vi "Histerisis.vi"() -> ()   [LabVIEW 2020]
uses:
  <vilib>/numeric/Random Number (Range) U64.vi
  <vilib>/numeric/sub_Random U32.vi
panel:
  in  "stop":bool
  out "XY Graph 2":cluster{i32, "number":u64}[](graph)
  in  "Minimo 2":u64
  in  "Maximo 2":u64
  out "Señal 2":bool
  out "Numero 2":u64
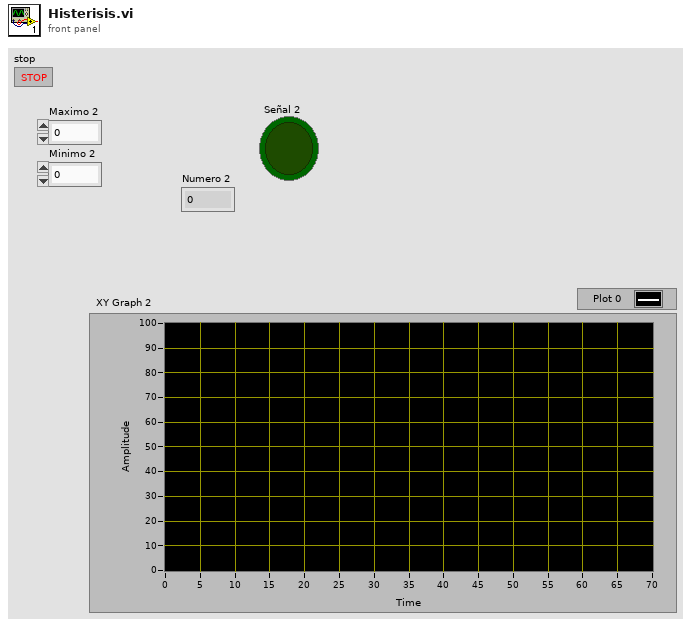
[diagram p1: front panel]
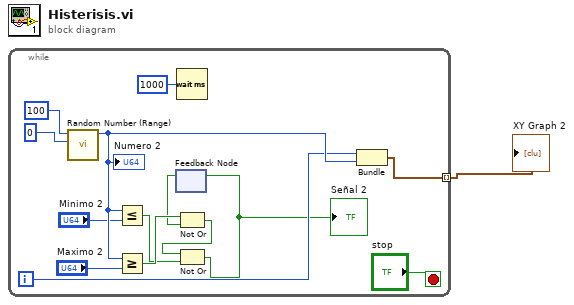
[diagram p0: block diagram]
diagram:
  n1 = while {
    tunnel: [w10] -> w1 mode=indexing
    i -> [w9]
    stop <- "stop" stop-if-true
    n2 = call-poly <vilib>:"Random Number (Range).vi"("lower bound (0)"=u64 0, "upper bound (100)"=u64 100) -> ("number"=w15:u64)  [unwired: 9 in]
    "Numero 2" <- w15
    n3 = Less Or Equal?(x=w15, y="Minimo 2") -> (x <= y?=w5:bool)
    n4 = Greater Or Equal?(x=w15, y="Maximo 2") -> (x >= y?=w6:bool)
    n5 = feedback #1() -> (w3:bool)  [unwired: 1 in]
    n6 = Wait (ms)(milliseconds to wait=u32 1000) -> ()  [unwired: 1 out]
    n7 = Not Or(1:w3, 2:w6) -> (0:w4:bool)
    n8 = Not Or(1:w5, 2:w4) -> (0:w2:bool)
    "Señal 2" <- w2
    n9 = feedback-in #1(w2) -> ()
    n10 = Bundle(w9, "number"=w15) -> (w10:cluster{i32, "number":u64})  [unwired: 1 in]
  }
  "XY Graph 2" <- w1
